vi "clockwise Reverse Logic.vi"(8 "error in (no error)":errorcluster, 11 "Programming Logic in":refnum<class "Programming Logic.lvclass">) -> (0 "error out":errorcluster, 3 "Programming Logic out":refnum<class "Programming Logic.lvclass">)   [LabVIEW 2014, in "Files Library.lvlib" / "Programming Logic.lvclass"]
uses:
  Programming Logic.lvclass
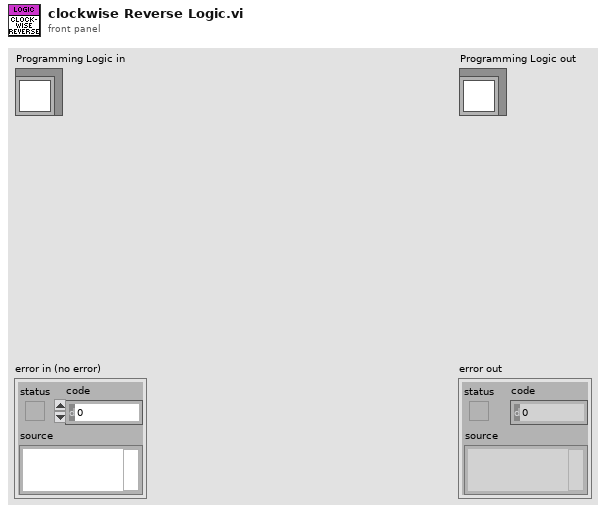
[diagram p1: front panel]
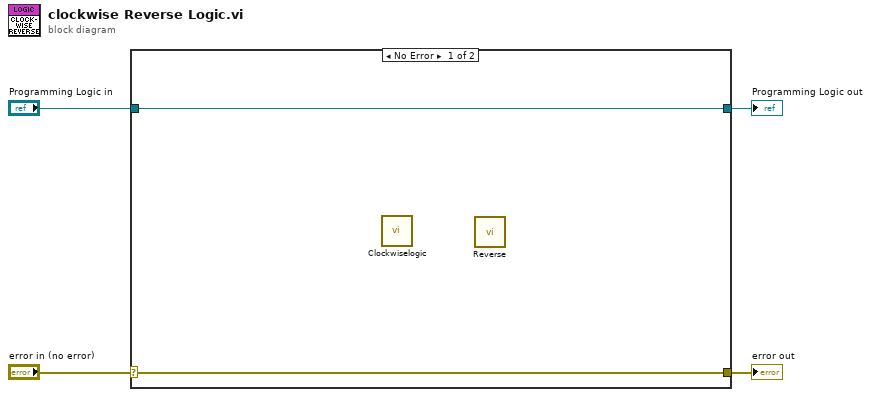
[diagram p0: block diagram]
diagram:
  n1 = case shown="No Error" "error in (no error)" {
    selector: "error in (no error)" -> [w5 w8]
    tunnel: [w5 w8] -> w3
    tunnel: [w6 w7] -> w1
    tunnel: "Programming Logic in" -> [w6 w7]
    frame No Error {
      n2 = call-dynamic "Clockwiselogic.vi"() -> ()  [unwired: 10 in, 2 out]
      n3 = call-dynamic "Reverse.vi"() -> ()  [unwired: 10 in, 2 out]
    }
    frame Error {
    }
  }
  "error out" <- w3
  "Programming Logic out" <- w1
